vi "InitializeParallelInstrument.vi"(8 "error in (no error)":errorcluster) -> (0 "error out":errorcluster, 3 "Parallel Instrument OUT":refnum<visa-resource-name>)   [LabVIEW 2017, in "Thermal Shock.lvlib"]
uses:
  Thermal Shock.lvlib
  <vilib>/Instr/_visa.llb/VISA Configure Serial Port (Instr).vi
panel:
  in  "Parallel Instrument IN":refnum<visa-resource-name>="LPT1"
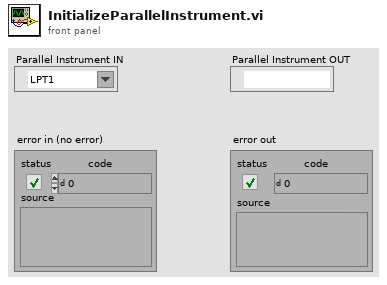
[diagram p1: front panel]
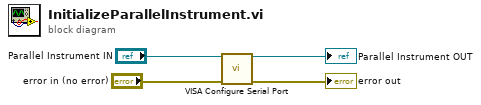
[diagram p0: block diagram]
diagram:
  n1 = call-poly "VISA Configure Serial Port"("VISA resource name"="Parallel Instrument IN", "error in (no error)"="error in (no error)") -> ("VISA resource name out"=→"Parallel Instrument OUT":refnum<visa-resource-name>, "error out"=→"error out":errorcluster)  [unwired: 12 in]
